vi "ex15-3.vi"() -> ()   [LabVIEW 2013]
uses:
  <vilib>/NXT/Block Support/NXT_OutputPort.ctl
  <vilib>/University of Leeds/Kinesthesia Toolkit for Microsoft Kinect/_Polymorphic Configure/Event-Skeleton and Video.vi
  <vilib>/University of Leeds/Kinesthesia Toolkit for Microsoft Kinect/_Polymorphic Close/Close-Skeleton and Video.vi
  <vilib>/University of Leeds/Kinesthesia Toolkit for Microsoft Kinect/_Polymorphic Read/Read-Skeleton and Video.vi
  <vilib>/NXT/NXTIO Xnodes/NXTIONodeSubVIs/NXTMoveMotors.vi
  <vilib>/NXT/Subs/LVHSConnector.ctl
  <vilib>/NXT/NXTIO Xnodes/AddressXNode/NXTIOAddress.xnode
  <vilib>/express/express arith-compare/Formula/XNode/ExpressFormulaBlockNode.xnode
  <vilib>/NXT/NXTIO Xnodes/NXTIOXNode/NXTIO.xnode
  <vilib>/NXT/LegoClasses/BrickReference/BrickReference.lvclass
panel:
  in  "stop":bool
  out "Left Go Forward":bool
  out "Left Speed":dbl(knob) scale=0.0..100.0
  out "Left Hand Angle":dbl
  out "Right Go Forward":bool
  out "Right Speed":dbl(knob) scale=0.0..100.0
  out "Right Hand Angle":dbl
  out "new picture":picture
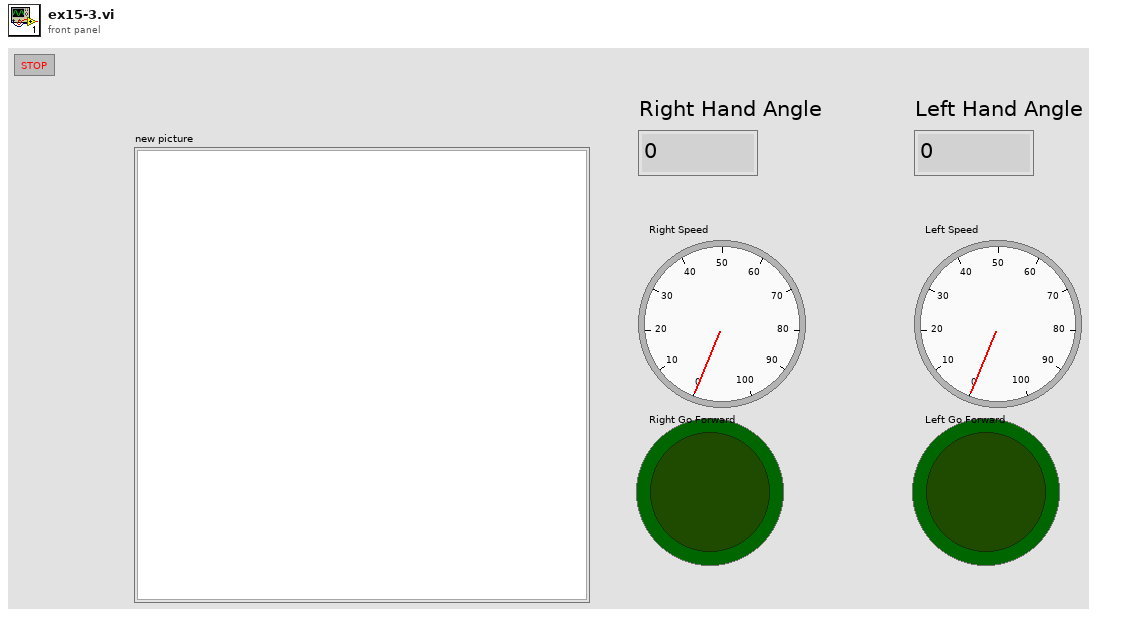
[diagram p1: front panel]
types:
  T1 = enum16{"hip centre", "spine", "shoulder centre", "head", "shoulder left", "elbow left", "wrist left", "hand left", "shoulder right", "elbow right", "wrist right", "hand right", "hip left", "knee left", "ankle left", "foot left", "hip right", "knee right", "ankle right", "foot right"}
  T2 = cluster{cluster{"reference out":refnum<k24>, "KinectSensors":refnum<k24>}, "get_Item":refnum<k24>}
  T3 = cluster{"reference out":refnum<k24>, "KinectSensors":refnum<k24>, "SkeletonStream":refnum<k24>, "ColorStream":refnum<k24>, refnum<k24>[], "get_Item":refnum<k24>}
  T4 = typedef "NXT_OutputPort.ctl" = u8
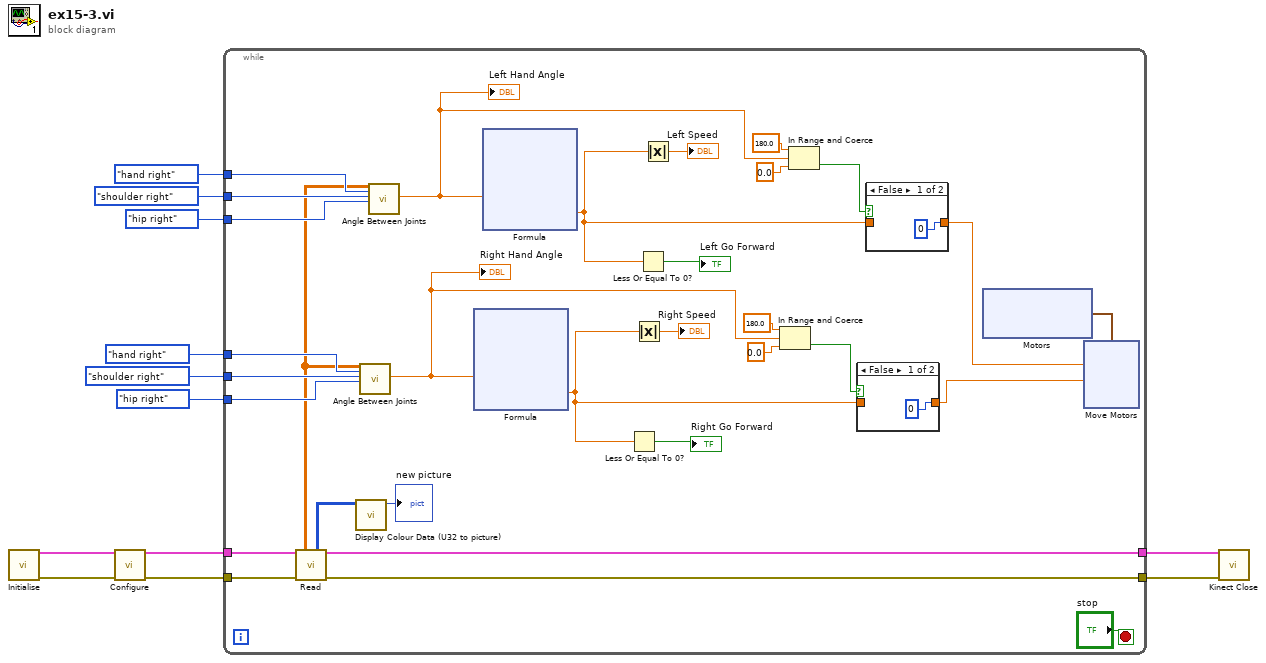
[diagram p0: block diagram]
diagram:
  n1 = call <vilib>:"Initialise.vi"() -> ("Kinect References out"=w12:T2, "error out"=w9:errorcluster)  [unwired: 14 in]
  n2 = call-poly <vilib>:"Configure.vi"("Kinect References in"=w12, "error in"=w9) -> ("Kinect References out"=w11:T3, "error out"=w8:errorcluster)  [unwired: 12 in]
  n3 = while {
    tunnel: w11 -> [w43]
    tunnel: [w42] -> w10
    tunnel: w8 -> [w41]
    tunnel: [w40] -> w7
    tunnel: T1."shoulder right" ("Joint 2") -> [w37]
    tunnel: T1."hip right" ("Joint 3") -> [w36]
    tunnel: T1."hand right" ("Joint 1") -> [w35]
    tunnel: T1."shoulder right" ("Joint 2") -> [w25]
    tunnel: T1."hip right" ("Joint 3") -> [w24]
    tunnel: T1."hand right" ("Joint 1") -> [w23]
    stop <- "stop" stop-if-true
    n4 = call-poly <vilib>:"Read.vi"("Kinect References in"=w43, "error in (no error)"=w41) -> ("Primary Skeleton Array"=w13:dbl[][], "Colour output array (U24, RGB)"=w39:u32[][], "Kinect References out"=w42:T3, "error out"=w40:errorcluster)  [unwired: 9 in, 1 out]
    n5 = call <vilib>:"Display Colour Data (U32 to picture).vi"("Colour output array (U24, RGB)"=w39) -> ("new picture"=→"new picture":picture)  [unwired: 10 in]
    n6 = call <vilib>:"Angle Between Joints.vi"("Array of Joint Positions"=w13, "Joint 1"=w35, "Joint 2"=w37, "Joint 3"=w36) -> ("Angle Between Joints (degrees)"=w32:dbl)  [unwired: 10 in, 5 out]
    "Right Hand Angle" <- w32
    n7 = call <vilib>:"Angle Between Joints.vi"("Array of Joint Positions"=w13, "Joint 1"=w23, "Joint 2"=w25, "Joint 3"=w24) -> ("Angle Between Joints (degrees)"=w20:dbl)  [unwired: 10 in, 5 out]
    "Left Hand Angle" <- w20
    n8 = xnode "Formula"("X1"=w32) -> ("Result"=w28:dbl)  [unwired: 1 in, 1 out]
    n9 = xnode "Formula"("X1"=w20) -> ("Result"=w16:dbl)  [unwired: 1 in, 1 out]
    n10 = Less Or Equal To 0?(x=w28) -> (x <= 0?=→"Right Go Forward":bool)
    n11 = Absolute Value(x=w28) -> (abs(x)=→"Right Speed":dbl)
    n12 = Less Or Equal To 0?(x=w16) -> (x <= 0?=→"Left Go Forward":bool)
    n13 = Absolute Value(x=w16) -> (abs(x)=→"Left Speed":dbl)
    n14 = In Range and Coerce(upper limit=180.0, x=w32, lower limit=0.0) -> (In Range?=w29:bool)  [unwired: 1 out]
    n15 = In Range and Coerce(upper limit=180.0, x=w20, lower limit=0.0) -> (In Range?=w17:bool)  [unwired: 1 out]
    n16 = case shown="False" w29 {
      tunnel: [0 w64] -> w26
      tunnel: w28 -> [_ w64]
      frame False {
      }
      frame True {
      }
    }
    n17 = case shown="False" w17 {
      tunnel: [0 w45] -> w15
      tunnel: w16 -> [_ w45]
      frame False {
      }
      frame True {
      }
    }
    n18 = xnode "Motors"() -> ("Motor"=w27:cluster{"Port":T4, "Port":T4})
    n19 = xnode "Move Motors"("Power/Speed 2"=w26, "Power/Speed 1"=w15, "Motors"=w27) -> ()  [unwired: 1 in, 1 out]
  }
  n20 = call-poly <vilib>:"Kinect Close.vi"("Kinect References in"=w10, "error in"=w7) -> ()  [unwired: 13 in, 1 out]
